vi "Print Console.vi"() -> ()   [LabVIEW 2010]
doc: "This print queue console simulates the control of print job submissions and monitors the status of the print jobs being processed."
uses:
  Print Indicators.ctl
  Print Processing States.ctl
panel:
  out "Print Indicators":T1={"Waiting"=TRUE, "Initializing"=FALSE, "Printing"=FALSE, "Job Number"=0}
  out "Queued Print Jobs":i32(slide) scale=0.0..25.0
  in  "Queue Event":bool
  in  "Stop":bool
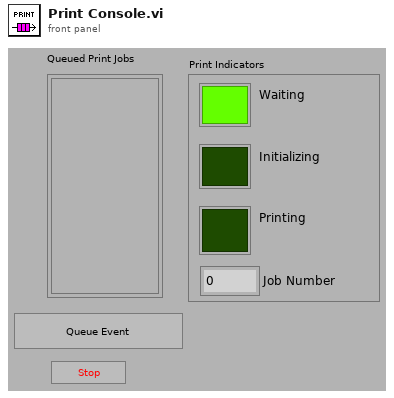
[diagram p1: front panel]
types:
  T1 = typedef "Print Indicators.ctl" = cluster{"Waiting":bool, "Initializing":bool, "Printing":bool, "Job Number":i32}
  T2 = typedef "Print Processing States.ctl" = enum16{"Wait", "Initialize Setup", "Setup", "Initialize Print", "Print", "Shutdown"}
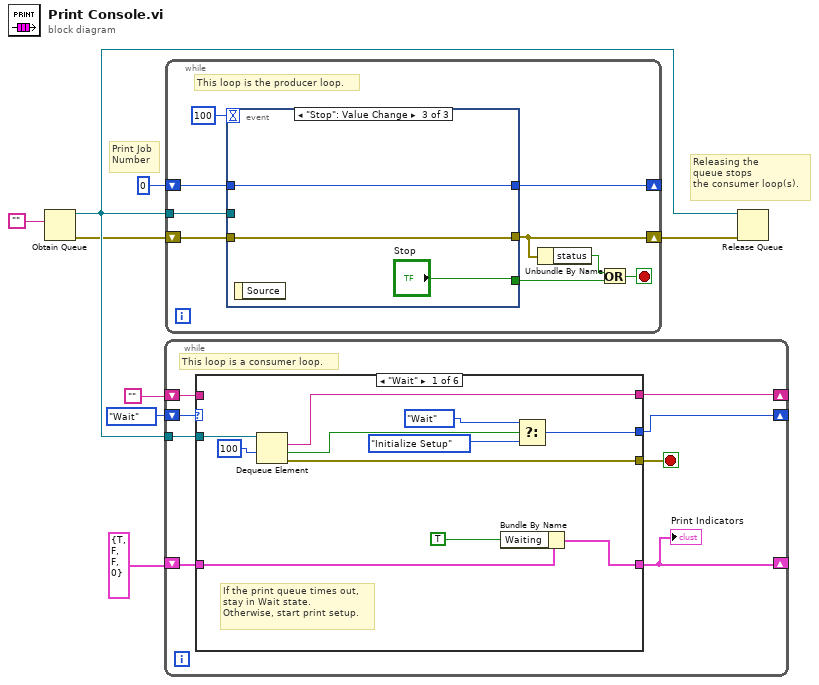
[diagram p0: block diagram]
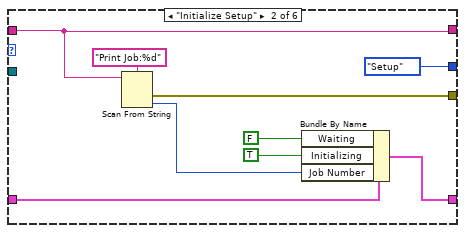
[diagram p2: hidden frame]
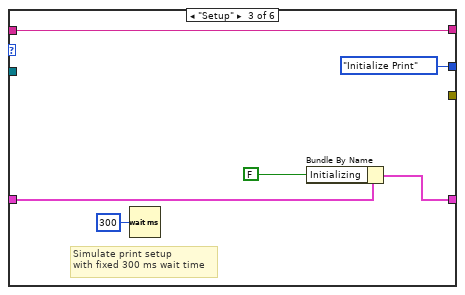
[diagram p3: hidden frame]
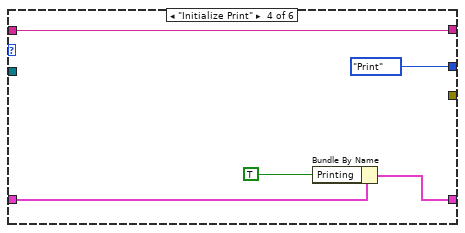
[diagram p4: hidden frame]
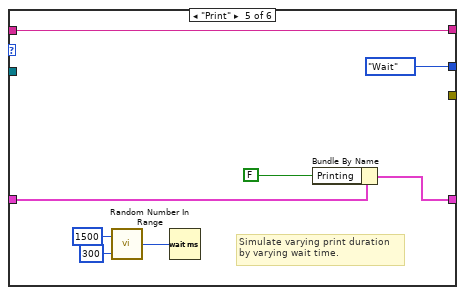
[diagram p5: hidden frame]
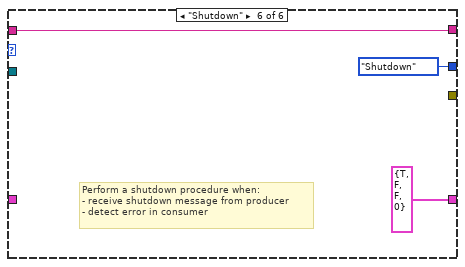
[diagram p6: hidden frame]
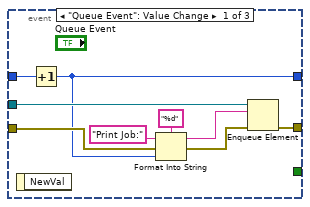
[diagram p7: hidden frame]
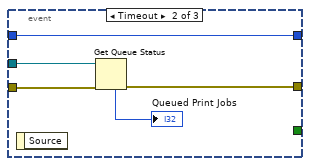
[diagram p8: hidden frame]
diagram:
  # "Print Job\nNumber"
  # "Releasing the\nqueue stops\nthe consumer loop(s)."
  n1 = Obtain Queue(element data type="") -> (queue out=w7:refnum<queue>, error out=w1:errorcluster)  [unwired: 4 in, 1 out]
  n2 = while {
    tunnel: w7 -> [w16]
    shift-right: [w10] -> _
    shift-left: Print_Processing_States."Wait" ("Enum") -> [w15]
    shift-right: [w13] -> _
    shift-left: T1 {"Waiting"=TRUE, "Initializing"=FALSE, "Printing"=FALSE, "Job Number"=0} ("Print LEDs") -> [w14]
    shift-right: [w11] -> _
    shift-left: "" -> [w12]
    stop <- w9 stop-if-true
    # "This loop is a consumer loop."
    n3 = case shown="\"Wait\"" w15 {
      tunnel: w16 -> [w27 _ _ _ _ _]
      tunnel: [w26 w28 _ _ _ _] -> w9
      tunnel: w14 -> [w21 w35 w41 w46 w54 _]
      tunnel: [w20 w34 w40 w45 w53 T1 {"Waiting"=TRUE, "Initializing"=FALSE, "Printing"=FALSE, "Job Number"=0} ("Print LEDs")] -> w13
      tunnel: [w18 Print_Processing_States."Setup" ("Enum") Print_Processing_States."Initialize Print" ("Enum") Print_Processing_States."Print" ("Enum") Print_Processing_States."Wait" ("Enum") Print_Processing_States."Shutdown" ("Enum")] -> w10
      tunnel: [w17 w31 w37 w43 w48 w56] -> w11
      tunnel: w12 -> [_ w31 w37 w43 w48 w56]
      frame "Wait" {
        # "If the print queue times out, \nstay in Wait state.\nOtherwise, start print setup."
        n4 = Dequeue Element(queue=w27, timeout in ms (-1)=100) -> (element=w17:string, timed out?=w19:bool, error out=w26:errorcluster)  [unwired: 1 in, 1 out]
        n5 = Bundle By Name(cluster=w21, "Waiting"=TRUE ("Waiting for\nnew job...")) -> (w20:T1)
        n6 = Select(t=Print_Processing_States."Wait" ("Enum"), s=w19, f=Print_Processing_States."Initialize Setup" ("Enum")) -> (s? t:f=w18:T2)
      }
      frame "Initialize Setup" {
        n7 = Scan From String(format string="Print Job:%d", input string=w31) -> (error out=w28:errorcluster, output 1=w29:i32)  [unwired: 3 in, 2 out]
        n8 = Bundle By Name(cluster=w35, "Waiting"=FALSE ("Waiting for\nnew job..."), "Initializing"=TRUE ("Waiting for\nnew job..."), "Job Number"=w29) -> (w34:T1)
      }
      frame "Setup" {
        # "Simulate print setup\nwith fixed 300 ms wait time"
        n9 = Wait (ms)(milliseconds to wait=u32 300) -> ()  [unwired: 1 out]
        n10 = Bundle By Name(cluster=w41, "Initializing"=FALSE ("Waiting for\nnew job...")) -> (w40:T1)
      }
      frame "Initialize Print" {
        n11 = Bundle By Name(cluster=w46, "Printing"=TRUE ("Waiting for\nnew job...")) -> (w45:T1)
      }
      frame "Print" {
        # "Simulate varying print duration\nby varying wait time."
        n12 = call "Random Number In Range.vi"("Lower Limit"=u32 300, "Upper Limit"=u32 1500) -> ("Random #"=w49:u32)
        n13 = Wait (ms)(milliseconds to wait=w49) -> ()  [unwired: 1 out]
        n14 = Bundle By Name(cluster=w54, "Printing"=FALSE ("Waiting for\nnew job...")) -> (w53:T1)
      }
      frame "Shutdown" {
        # "Perform a shutdown procedure when:\n- receive shutdown message from producer\n- detect error in consumer"
      }
    }
    "Print Indicators" <- w13
  }
  n15 = while {
    tunnel: w7 -> [w67]
    shift-right: [w61] -> _
    shift-left: 0 -> [w62]
    shift-right: [w60] -> w2
    shift-left: w1 -> [w59]
    stop <- w65 stop-if-true
    # "This loop is the producer loop."
    n16 = event shown="[2] \"Stop\": Value Change" {
      selector: _ -> [_ _ _]
      dyn-events: _ -> [_ _ _]
      timeout: 100 -> [_ _ _]
      tunnel: w67 -> [w76 w79 _]
      tunnel: w59 -> [w74 w80 w82]
      tunnel: [w75 w78 w82] -> w60
      tunnel: [_ _ "Stop"] -> w66
      tunnel: w62 -> [w70 w77 w83]
      tunnel: [w68 w77 w83] -> w61
      event "Queue Event": Value Change {
        n17 = event-data() -> ()  [unwired: 1 in, 1 out]
        n18 = Increment(x=w70) -> (x+1=w68:i32)
        n19 = Format Into String(format string="%d", initial string="Print Job:", error in=w74, w68) -> (resulting string=w69:string, error out=w73:errorcluster)
        n20 = Enqueue Element(queue=w76, element=w69, error in (no error)=w73) -> (error out=w75:errorcluster)  [unwired: 1 in, 2 out]
      }
      event Timeout {
        n21 = event-data() -> ()  [unwired: 1 in, 1 out]
        n22 = Get Queue Status(queue=w79, error in (no error)=w80) -> (error out=w78:errorcluster, # elements in queue=→"Queued Print Jobs":i32)  [unwired: 1 in, 6 out]
      }
      event "Stop": Value Change {
        n23 = event-data() -> ()  [unwired: 1 in, 1 out]
      }
    }
    n24 = Unbundle By Name(w60) -> ("status"=w64:bool)
    n25 = Or(x=w64, y=w66) -> (x .or. y?=w65:bool)
  }
  n26 = Release Queue(queue=w7, error in (no error)=w2) -> ()  [unwired: 1 in, 3 out]
